vi "Add Padding & Length.vi"(11 "Data":u8[](array[numeric])) -> (3 "Padded Data":u8[](array[numeric]) format="%08b", 5 "Blocks":i32)   [LabVIEW 2020, in "Crypto.lvlib" / "MD5.lvclass"]
uses:
  MD5.lvclass
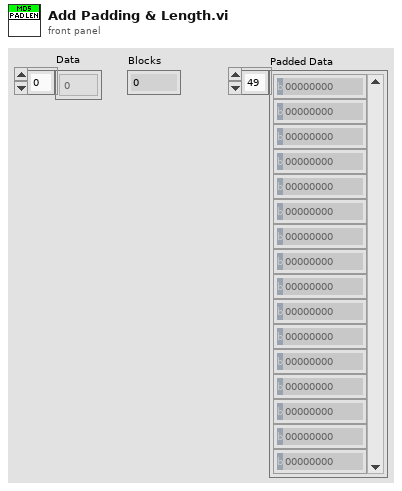
[diagram p1: front panel]
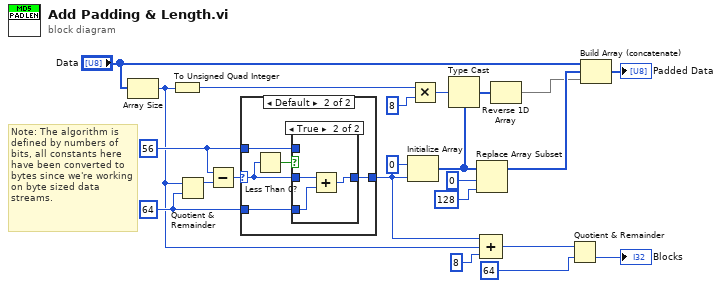
[diagram p0: block diagram]
diagram:
  w20 = 56 ("x")
  w16 = 64 ("y")
  # "Note: The algorithm is defined by numbers of bits, all constants here have been converted to bytes since we're working on byte sized data streams."
  n1 = Array Size(array="Data") -> (size(s)=w9:i32)
  n2 = To Unsigned Quad Integer(1:w9) -> (0:w12:u64)
  n3 = Quotient & Remainder(x=w9, y=w16) -> (x-y*floor(x/y)=w22:i32)  [unwired: 1 out]
  n4 = Subtract(x=w20, y=w22) -> (x-y=w21:i32)
  n5 = case shown="Default" w21 {
    selector: w21 -> [_ w27]
    tunnel: w20 -> [_ w26]
    tunnel: [w23 w25] -> w8
    tunnel: w16 -> [w23 w24]
    frame 0 {
    }
    frame Default {
      n6 = Less Than 0?(x=w27) -> (x < 0?=w28:bool)
      n7 = case shown="True" w28 {
        tunnel: w27 -> [w29 w30]
        tunnel: [w29 w32] -> w25
        tunnel: w26 -> [_ _]
        tunnel: w24 -> [_ w31]
        frame False {
        }
        frame True {
          n8 = Add(x=w30, y=w31) -> (x+y=w32:i32)
        }
      }
    }
  }
  n9 = Initialize Array(u8 0 ("element"), w8) -> (w10:u8[])
  n10 = Multiply(x=w12, y=u64 8) -> (x*y=w3:u64)
  n11 = Type Cast(type=w10, x=w3) -> (*(type *) &x=w11:u8[])
  n12 = Replace Array Subset(array=w10, new element=u8 128 ("new element/subarray"), index=0) -> (w14:u8[])
  n13 = Compound Arithmetic op=ADD(w8, w9, 8 ("value")) -> (w7:i32)
  n14 = Reverse 1D Array(array=w11) -> (reversed array=w1:u8[])
  n15 = Quotient & Remainder(x=w7, y=64) -> (floor(x/y)=→"Blocks":i32)  [unwired: 1 out]
  n16 = Build Array (concatenate)("Data", w14, w1) -> (→"Padded Data":u8[])
